vi "Correct Data.vi"(8 "error in":errorcluster, 10 "Data In":refnum<class "Data.lvclass">, 11 "Configurable Device in":refnum<class "Configurable Device.lvclass">) -> (0 "error out":errorcluster, 2 "Data Out":refnum<class "Data.lvclass">, 3 "Configurable Device out":refnum<class "Configurable Device.lvclass">)   [LabVIEW 2016, in "Configurable Device.lvclass"]
uses:
  Configurable Device.lvclass
  <vilib>/MSR Consulting, LLC/General Reuse/Data/Data.lvclass
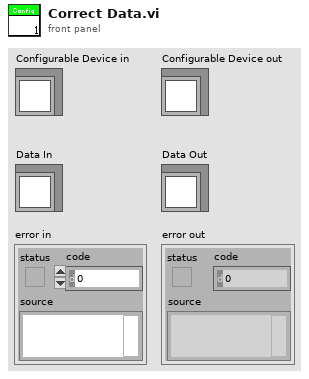
[diagram p1: front panel]
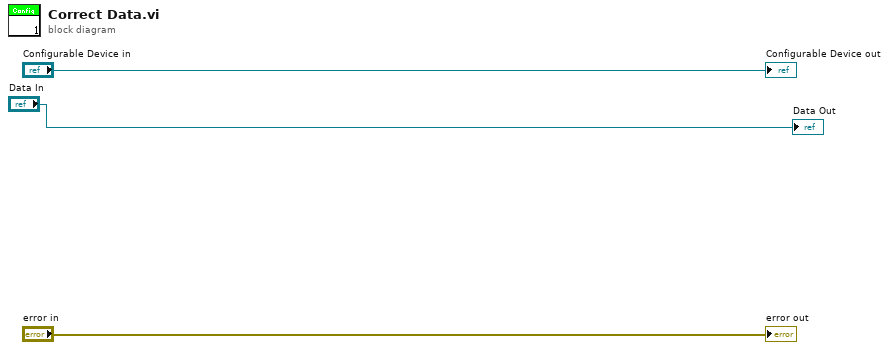
[diagram p0: block diagram]
diagram:
  "error out" <- "error in"
  "Configurable Device out" <- "Configurable Device in"
  "Data Out" <- "Data In"
